vi "Add Tool Menu Item.vi"(4 "Custom Shortcut":string, 6 "Name":string, 7 "Enabled?":bool, 8 "Error in":errorcluster, 9 "ID":string, 10 "Parent ID":string, 11 "Tools":refnum<vi>) -> (0 "Error Out":errorcluster)   [LabVIEW 2021, in "Seq Edit Quick Drop.lvlib"]
uses:
  Seq Edit Quick Drop.lvlib
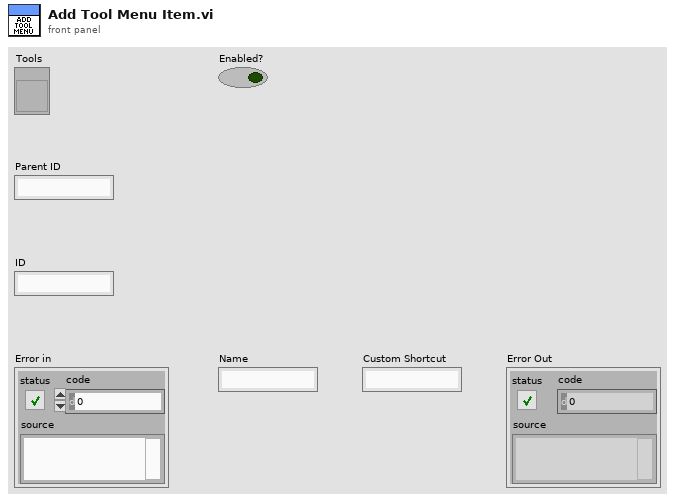
[diagram p1: front panel]
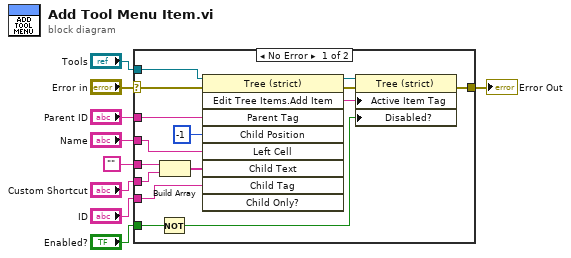
[diagram p0: block diagram]
diagram:
  n1 = case shown="No Error" "Error in" {
    selector: "Error in" -> [w11 w25]
    tunnel: "Name" -> [w24 _]
    tunnel: "Parent ID" -> [w23 _]
    tunnel: "Enabled?" -> [w22 _]
    tunnel: [w19 w25] -> w6
    tunnel: "Tools" -> [w16 _]
    tunnel: "ID" -> [w15 _]
    tunnel: "" -> [w14 _]
    tunnel: "Custom Shortcut" -> [w13 _]
    frame No Error {
      n2 = Not(x=w22) -> (.not. x?=w10:bool)
      n3 = Build Array(w14, w13) -> (w12:string[])
      n4 = invoke on="Invoke Node" class="Tree (strict)" method="Edit Tree Items.Add Item"(reference=w16, error in=w11, "Parent Tag"=w23, "Child Position"=-1, "Left Cell"=w24, "Child Text"=w12, "Child Tag"=w15) -> (reference out=w17:refnum<vi>, error out=w18:errorcluster, "Edit Tree Items:Add Item"=w21:string)  [unwired: 2 in, 6 out]
      n5 = property class="Tree (strict)"(reference=w17, error in=w18, "Active Item Tag"=w21, "Disabled?"=w10) -> (error out=w19:errorcluster)  [unwired: 1 out]
    }
    frame Error {
    }
  }
  "Error Out" <- w6
